vi "Cleanup.vi"(8 "error in (no error)":errorcluster, 11 "NodeRef In":refnum<data-value>) -> (0 "error out":errorcluster)   [LabVIEW 2020, in "PicoG-ParserLexer.lvlib" / "Node.lvclass"]
uses:
  Node.lvclass
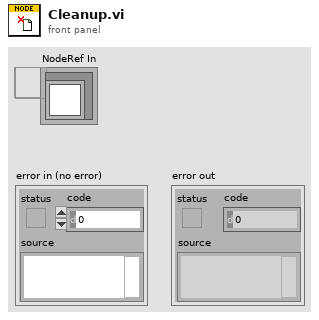
[diagram p1: front panel]
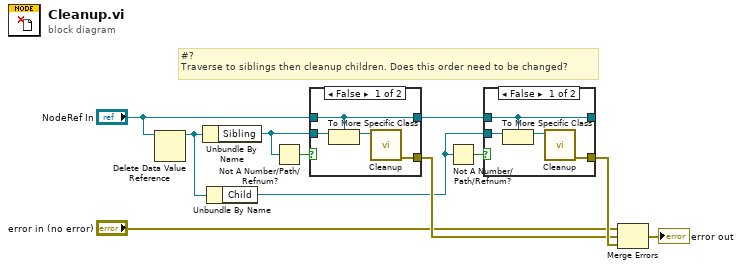
[diagram p0: block diagram]
diagram:
  # "#?\nTraverse to siblings then cleanup children. Does this order need to be changed?"
  n1 = Delete Data Value Reference(data value reference="NodeRef In") -> (data value=w6:refnum<class "Node.lvclass">)  [unwired: 1 in, 1 out]
  n2 = Unbundle By Name(w6) -> ("Sibling"=w8:refnum<data-value>)
  n3 = Unbundle By Name(w6) -> ("Child"=w4:refnum<data-value>)
  n4 = Not A Number/Path/Refnum?(number/path/refnum=w8) -> (NaN/Path/Refnum?=w9:bool)
  n5 = case shown="False" w9 {
    tunnel: w8 -> [w15 _]
    tunnel: "NodeRef In" -> [w12 w16]
    tunnel: [w13 _] -> w10
    tunnel: [w12 w16] -> w3
    frame False {
      n6 = To More Specific Class(target class=w12, reference=w15) -> (specific class reference=w14:refnum<data-value>)  [unwired: 1 in, 1 out]
      n7 = call "Cleanup.vi"("NodeRef In"=w14) -> ("error out"=w13:errorcluster)  [unwired: 10 in]
    }
    frame True {
    }
  }
  n8 = Not A Number/Path/Refnum?(number/path/refnum=w4) -> (NaN/Path/Refnum?=w5:bool)
  n9 = case shown="False" w5 {
    tunnel: w4 -> [w20 _]
    tunnel: w3 -> [w17 w21]
    tunnel: [w18 _] -> w11
    tunnel: [w17 w21] -> _
    frame False {
      n10 = To More Specific Class(target class=w17, reference=w20) -> (specific class reference=w19:refnum<data-value>)  [unwired: 1 in, 1 out]
      n11 = call "Cleanup.vi"("NodeRef In"=w19) -> ("error out"=w18:errorcluster)  [unwired: 10 in]
    }
    frame True {
    }
  }
  n12 = Merge Errors("error in (no error)", w10, w11) -> (→"error out":errorcluster)
